vi "Tarea 12.vi"() -> ()   [LabVIEW 2019]
uses:
  Student Material/Student Material/Module 3/Exercise 12/Controls/CLD 12 Data Cluster.ctl
  Student Material/Student Material/Module 3/Exercise 12/Controls/CLD 12 Sequencer Enum.ctl
  Student Material/Student Material/Module 3/Exercise 12/CLD3 Timer/CLD3 FGV Mode.ctl
panel:
  in  "Start":bool
  out "Switch 3":bool
  out "Switch 2":bool
  out "Switch 1":bool
  out "Time Elapsed":dbl
  in  "Stop Button":bool
  out "Current Time Target":dbl
  in  "error in (no error)":errorcluster
  out "error out":errorcluster
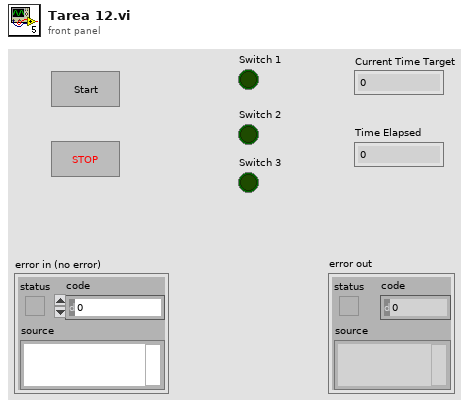
[diagram p1: front panel]
types:
  T1 = typedef "CLD 12 Data Cluster.ctl" = cluster{"Command":T2, "Time Value":dbl, "Boolean":bool, "Boolean 2":bool, "Boolean 3":bool}
  T2 = typedef "CLD 12 Sequencer Enum.ctl" = enum16{"Initialize", "SetTime", "RunState1", "Runstate2", "Idle", "Start"}
  T3 = typedef "CLD3 FGV Mode.ctl" = enum16{"Start Timer", "Reset Timer", "Read Time", "Pause", "Resume"}
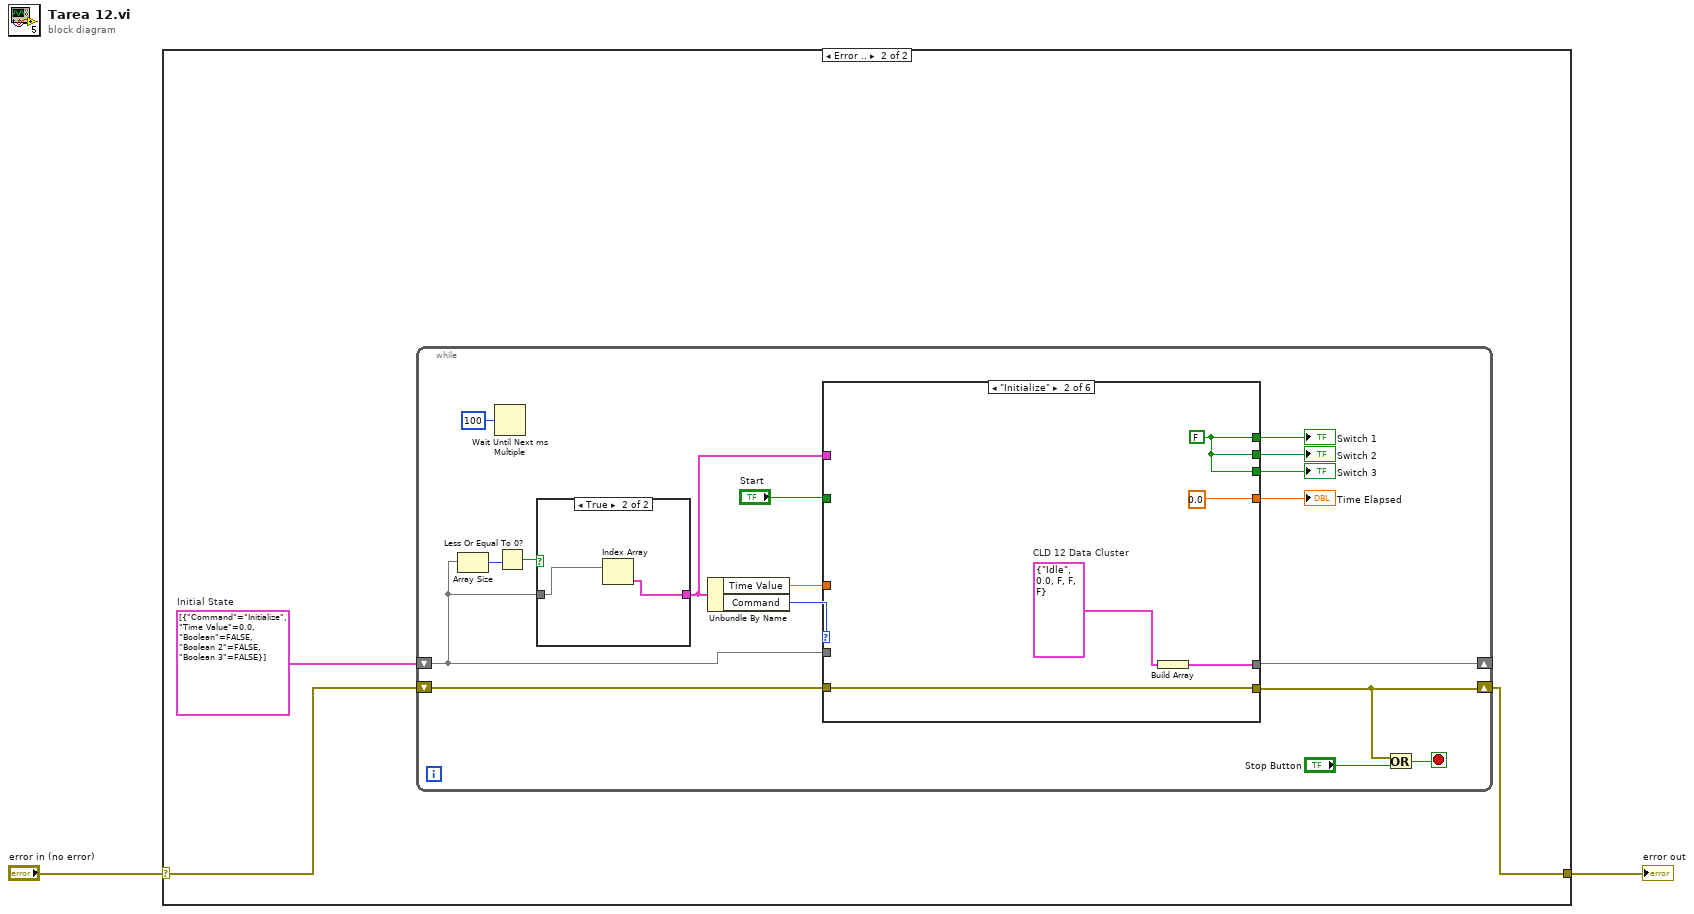
[diagram p0: block diagram]
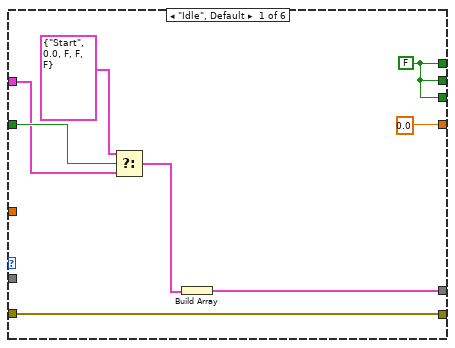
[diagram p3: hidden frame]
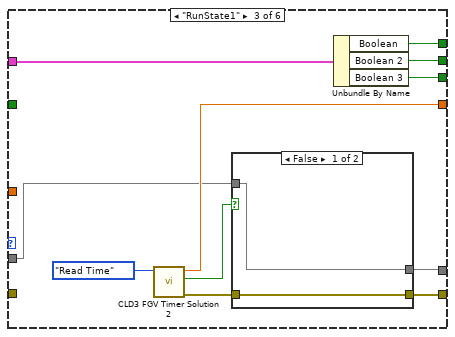
[diagram p4: hidden frame]
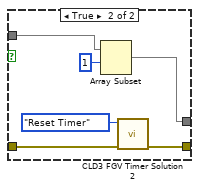
[diagram p5: hidden frame]
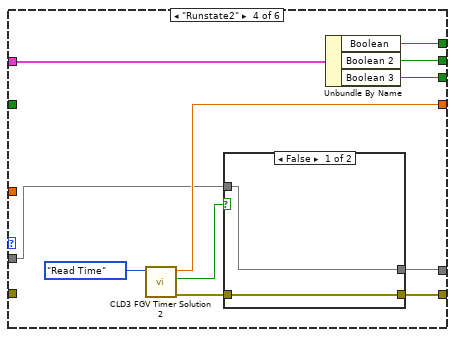
[diagram p6: hidden frame]
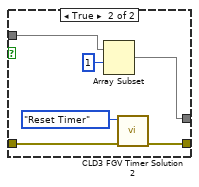
[diagram p7: hidden frame]
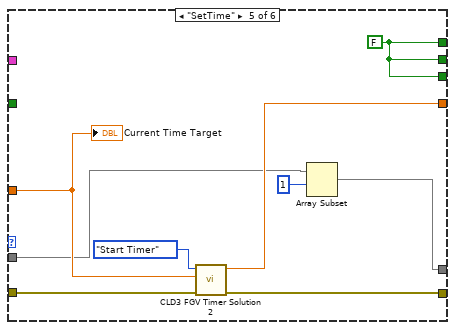
[diagram p8: hidden frame]
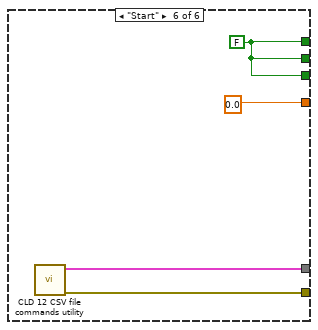
[diagram p9: hidden frame]
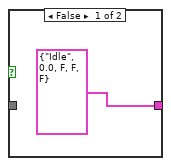
[diagram p10: hidden frame]
diagram:
  n1 = case shown="Error .." "error in (no error)" {
    selector: "error in (no error)" -> [w3 w6]
    tunnel: [w3 w5] -> w1
    frame No Error {
    }
    frame Error {
      w4 = T1[] [{"Command"=enum."Initialize", "Time Value"=0.0, "Boolean"=FALSE, "Boolean 2"=FALSE, "Boolean 3"=FALSE}]  # Initial State
      n2 = while {
        shift-right: [w9] -> w5
        shift-left: w6 -> [w12]
        shift-right: [w13] -> _
        shift-left: w4 -> [w7]
        stop <- w8 stop-if-true
        n3 = Array Size(array=w7) -> (size(s)=w11:i32)
        n4 = Wait Until Next ms Multiple(millisecond multiple=u32 100) -> ()  [unwired: 1 out]
        n5 = Less Or Equal To 0?(x=w11) -> (x <= 0?=w10:bool)
        n6 = case shown="True" w10 {
          tunnel: [T1 {"Command"=enum."Idle", "Time Value"=0.0, "Boolean"=FALSE, "Boolean 2"=FALSE, "Boolean 3"=FALSE} ("CLD 12 Data Cluster") w89] -> w17
          tunnel: w7 -> [_ w90]
          frame False {
            # "Array empty. Force Idle"
          }
          frame True {
            # "Extract element 0 in \narray"
            n7 = Index Array(array=w90) -> (element=w89:T1)  [unwired: 1 in]
          }
        }
        n8 = Unbundle By Name(w17) -> ("Time Value"=w16:dbl, "Command"=w18:T2)
        n9 = case shown="\"Initialize\"" w18 {
          tunnel: [w24 w32 w40 w63 w82 w87] -> w9
          tunnel: [w31 w36 w45 w60 w83 w86] -> w22
          tunnel: [w31 w36 w44 w59 w83 w86] -> w21
          tunnel: [w31 w36 w43 w58 w83 w86] -> w20
          tunnel: [0.0 ("Elapsed Time (s.ss)") 0.0 ("Elapsed Time (s.ss)") w46 w61 w80 0.0 ("Elapsed Time (s.ss)")] -> w19
          tunnel: [w29 w35 w37 w57 w75 w85] -> w13
          tunnel: w17 -> [w27 _ w39 w62 _ _]
          tunnel: w16 -> [_ _ _ _ w78 _]
          tunnel: "Start" -> [w28 _ _ _ _ _]
          tunnel: w12 -> [w24 w32 _ _ w77 _]
          tunnel: w7 -> [_ _ w38 w56 w76 _]
          frame "Idle", Default {
            w31 = FALSE ("Boolean 1")
            n10 = Select(t=T1 {"Command"=enum."Start", "Time Value"=0.0, "Boolean"=FALSE, "Boolean 2"=FALSE, "Boolean 3"=FALSE}, s=w28, f=w27) -> (s? t:f=w26:T1)
            n11 = Build Array(w26) -> (w29:T1[])
          }
          frame "Initialize" {
            w36 = FALSE ("Boolean 1")
            w33 = T1 {"Command"=enum."Idle", "Time Value"=0.0, "Boolean"=FALSE, "Boolean 2"=FALSE, "Boolean 3"=FALSE}  # CLD 12 Data Cluster
            n12 = Build Array(w33) -> (w35:T1[])
          }
          frame "RunState1" {
            n13 = call "CLD3 FGV Timer Solution 2.vi"("Timer Mode"=CLD3_FGV_Mode."Read Time") -> ("Error Out"=w41:errorcluster, "Has Time Elapsed"=w42:bool, "Elapsed Time (s.ss)"=w46:dbl)  [unwired: 8 in]
            n14 = case shown="False" w42 {
              tunnel: w41 -> [w49 w55]
              tunnel: [w49 w54] -> w40
              tunnel: [w48 w51] -> w37
              tunnel: w38 -> [w48 w50]
              frame False {
              }
              frame True {
                n15 = Array Subset "Array Subset"(array=w50, index=1) -> (w51:T1[])  [unwired: 1 in]
                n16 = call "CLD3 FGV Timer Solution 2.vi"("Error In"=w55, "Timer Mode"=CLD3_FGV_Mode."Reset Timer") -> ("Error Out"=w54:errorcluster)  [unwired: 7 in, 2 out]
              }
            }
            n17 = Unbundle By Name(w39) -> ("Boolean"=w45:bool, "Boolean 2"=w44:bool, "Boolean 3"=w43:bool)
          }
          frame "Runstate2" {
            n18 = call "CLD3 FGV Timer Solution 2.vi"("Timer Mode"=CLD3_FGV_Mode."Read Time") -> ("Error Out"=w64:errorcluster, "Has Time Elapsed"=w65:bool, "Elapsed Time (s.ss)"=w61:dbl)  [unwired: 8 in]
            n19 = case shown="False" w65 {
              tunnel: w64 -> [w68 w74]
              tunnel: [w68 w73] -> w63
              tunnel: [w67 w70] -> w57
              tunnel: w56 -> [w67 w69]
              frame False {
              }
              frame True {
                n20 = Array Subset "Array Subset"(array=w69, index=1) -> (w70:T1[])  [unwired: 1 in]
                n21 = call "CLD3 FGV Timer Solution 2.vi"("Error In"=w74, "Timer Mode"=CLD3_FGV_Mode."Reset Timer") -> ("Error Out"=w73:errorcluster)  [unwired: 7 in, 2 out]
              }
            }
            n22 = Unbundle By Name(w62) -> ("Boolean"=w60:bool, "Boolean 2"=w59:bool, "Boolean 3"=w58:bool)
          }
          frame "SetTime" {
            w83 = FALSE ("Boolean 1")
            n23 = call "CLD3 FGV Timer Solution 2.vi"("Error In"=w77, "Time Target (s)"=w78, "Timer Mode"=CLD3_FGV_Mode."Start Timer") -> ("Error Out"=w82:errorcluster, "Elapsed Time (s.ss)"=w80:dbl)  [unwired: 6 in, 1 out]
            n24 = Array Subset "Array Subset"(array=w76, index=1) -> (w75:T1[])  [unwired: 1 in]
            "Current Time Target" <- w78
          }
          frame "Start" {
            w86 = FALSE ("Boolean 1")
            n25 = call "CLD 12 CSV file commands utility.vi"() -> ("Error Out"=w87:errorcluster, "Command Array Out"=w85:T1[])  [unwired: 10 in]
          }
        }
        "Time Elapsed" <- w19
        "Switch 1" <- w22
        "Switch 2" <- w21
        "Switch 3" <- w20
        n26 = Or(x=w9, y="Stop Button") -> (x .or. y?=w8:bool)
      }
    }
  }
  "error out" <- w1
